vi "Logging Message Loop.vi"(8 "error in (no error)":errorcluster, 10 "Data Queue":refnum<queue>, 11 "Message Queues":T1) -> (0 "error out":errorcluster)   [LabVIEW 2017, in "Logging.lvlib"]
doc: "The message loop subVI to handle messages pertaining to logging data."
uses:
  Logging.lvlib
  support/Message Queue/All Message Queues.ctl
  support/Message Queue/Message Cluster.ctl
  Logging Configuration.ctl
  Logging State.ctl
  <userlib>/Circular Buffer/Controls/Circular Buffer Operations.ctl
  <userlib>/Circular Buffer/Instance VIs/Circular Buffer(2D Wfm with Attributes).vi
  support/Message Queue/Enqueue Message (Single).vi
  <vilib>/Waveform/WDTOps.llb/WDT Number of Waveform Samples DBL.vi
  <vilib>/Utility/error.llb/Error Cluster From Error Code.vi
  <vilib>/ErrorRing/Error Ring.xnode
  support/Message Queue/Message Queue.lvlib
  <userlib>/Circular Buffer/Circular Buffer.lvlib
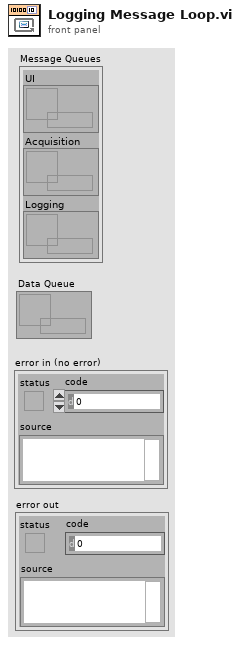
[diagram p1: front panel]
types:
  T1 = typedef "Message Queue.lvlib/All Message Queues.ctl" = cluster{"UI":refnum<queue>, "Acquisition":refnum<queue>, "Logging":refnum<queue>}
  T2 = typedef "Logging.lvlib/Logging State.ctl" = cluster{"State":enum16{"Logging", "Not Logging"}, "Samples to Save":u32, "Force Trigger":bool}
  T3 = typedef "Logging.lvlib/Logging Configuration.ctl" = cluster{"Log File Base Path":path, "Samples to Save":u32, "Trigger - Threshold":dbl, "Trigger - Channel":u32, "Always Log":bool, "External Trigger":bool, "External Trigger Armed":bool, "TDMS File Reference":refnum<k34>, "DAQVersion":string, "SWVersion":string, "CircSamples":u32, "BeepWhenComplete":bool, "ChannelConfig":string[][], "ActiveChannels":i32[], "Title":string, "Description":string, "ChannelNames":string[], "ResponseExtension":bool}
  T4 = typedef "Circular Buffer.lvlib/Circular Buffer Operations.ctl" = enum16{"Initialize", "Get Backlog", "Write", "Read (continuous)", "Read (most recent)", "Peak"}
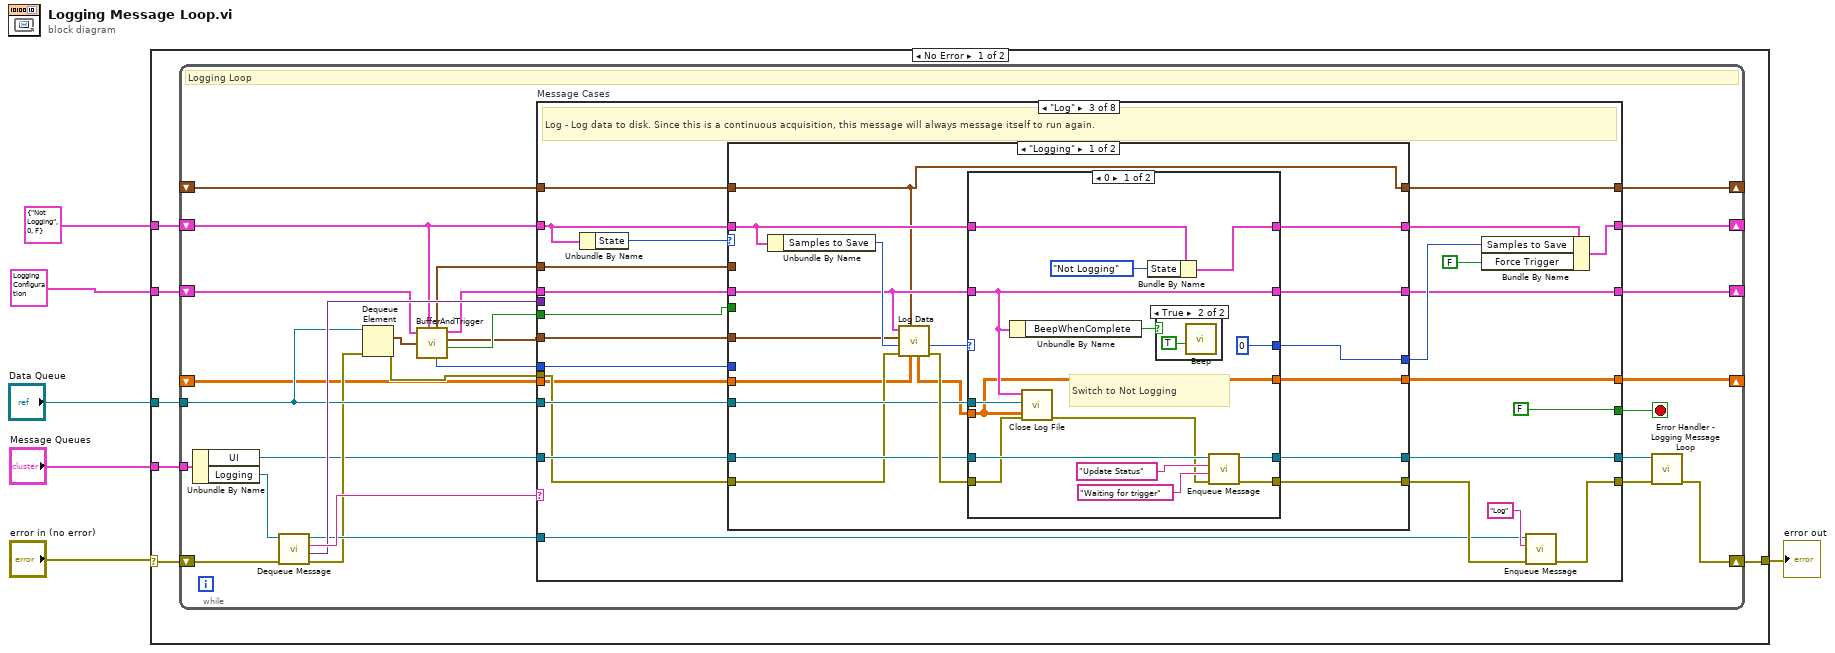
[diagram p0: block diagram]
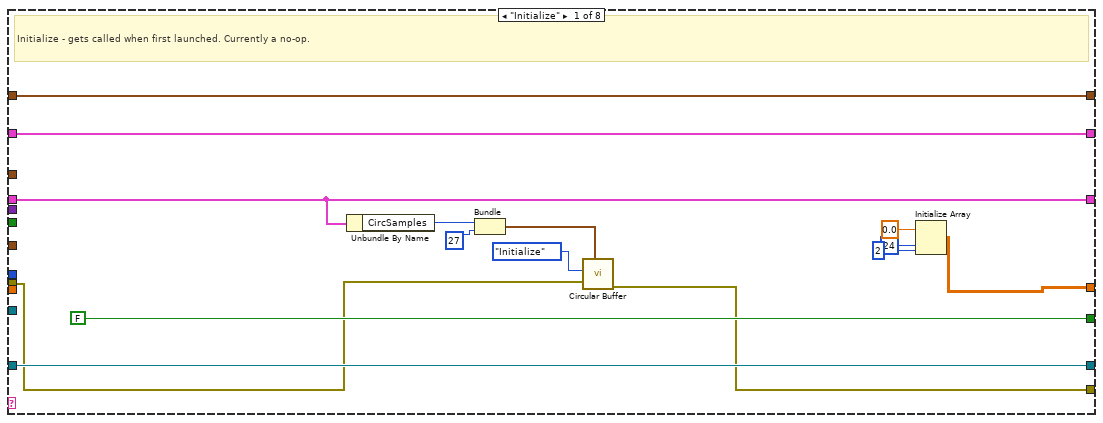
[diagram p2: hidden frame]
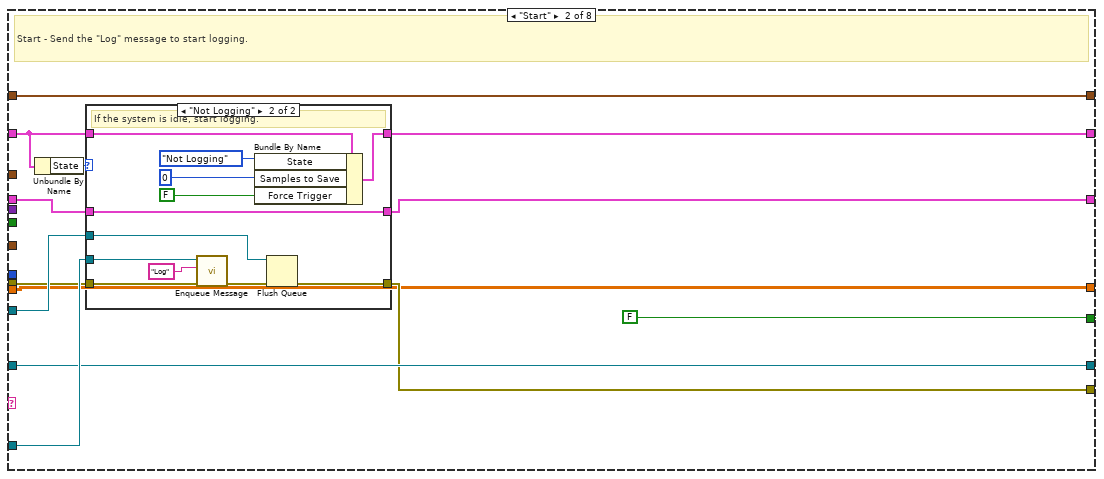
[diagram p3: hidden frame]
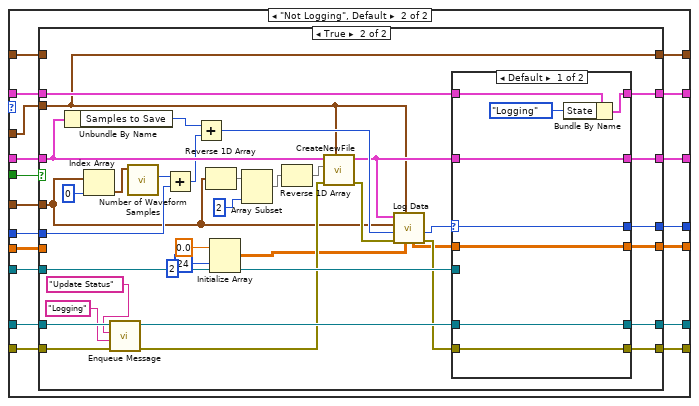
[diagram p7: hidden frame]
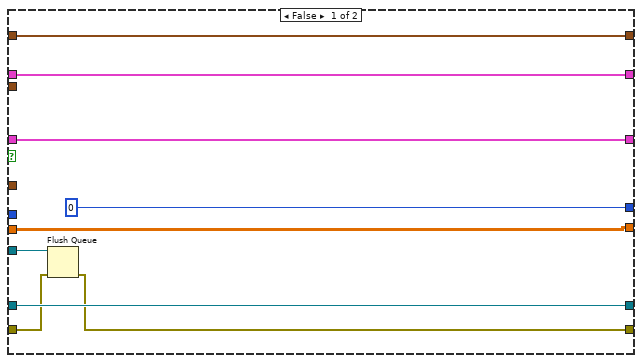
[diagram p8: hidden frame]
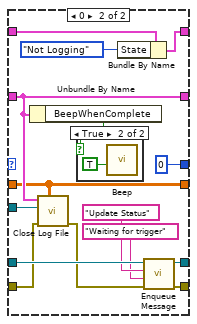
[diagram p9: hidden frame]
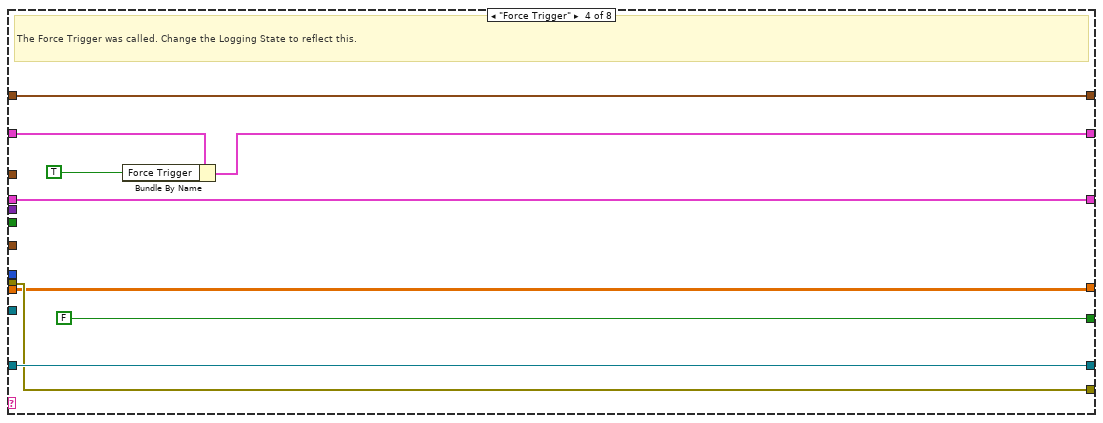
[diagram p11: hidden frame]
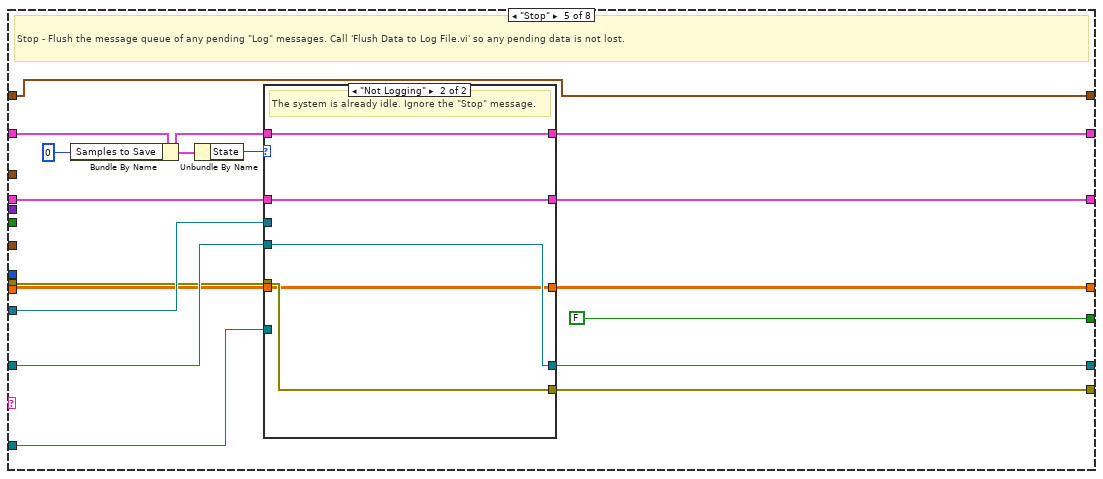
[diagram p12: hidden frame]
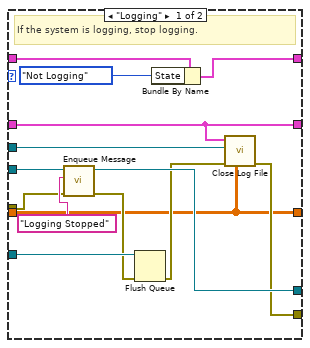
[diagram p13: hidden frame]
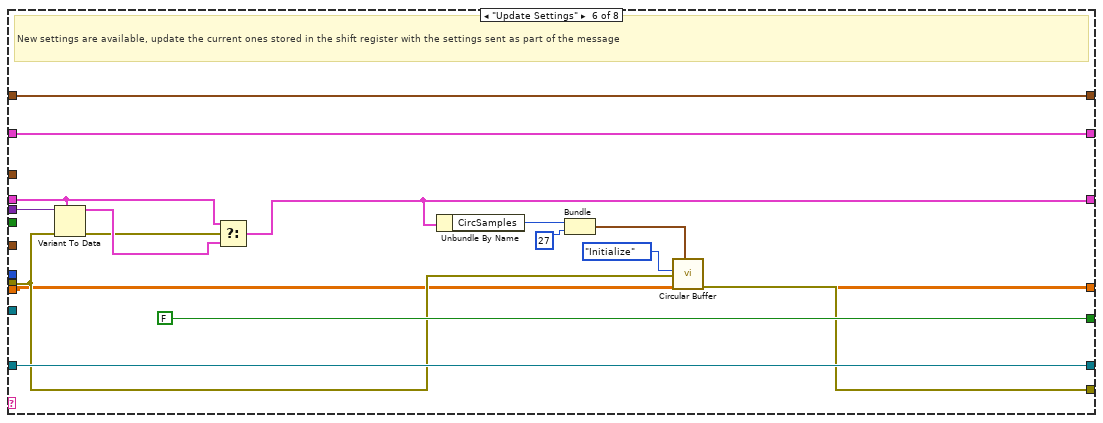
[diagram p14: hidden frame]
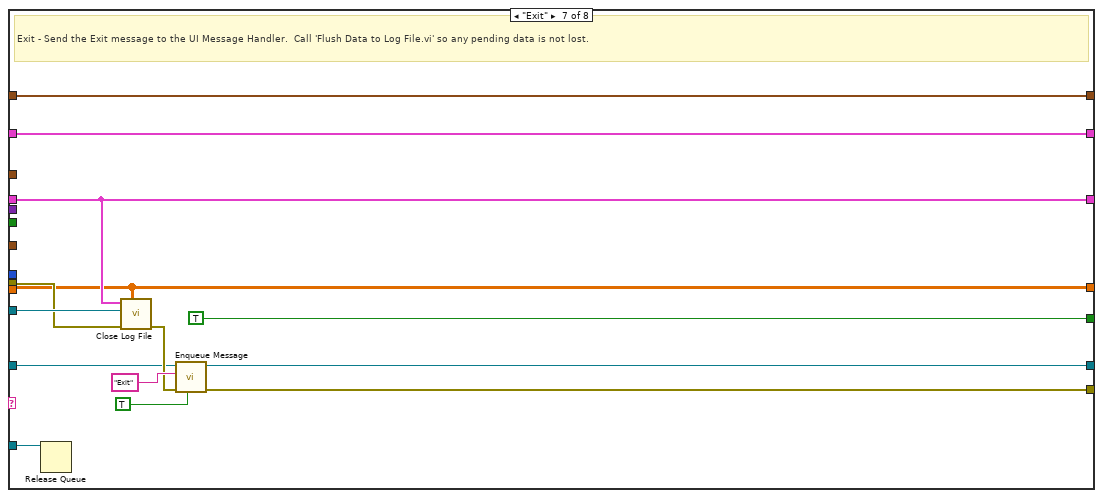
[diagram p15: hidden frame]
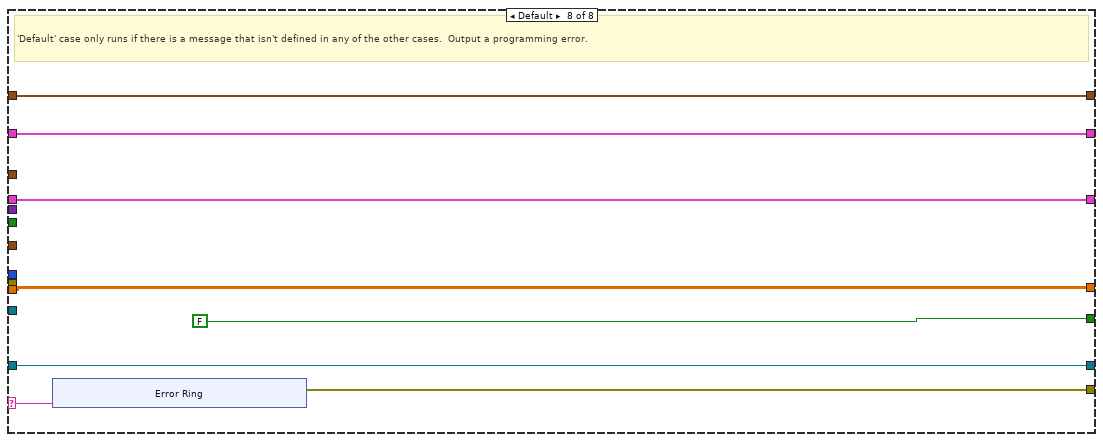
[diagram p16: hidden frame]
diagram:
  n1 = case shown="No Error" "error in (no error)" {
    selector: "error in (no error)" -> [w11 w327]
    tunnel: [w12 w327] -> w6
    tunnel: "Data Queue" -> [w10 _]
    tunnel: T2 {"State"=enum."Not Logging", "Samples to Save"=0, "Force Trigger"=FALSE} -> [w9 _]
    tunnel: T3 {"Log File Base Path"=path "", "Samples to Save"=0, "Trigger - Threshold"=0.0, "Trigger - Channel"=0, "Always Log"=FALSE, "External Trigger"=FALSE, "External Trigger Armed"=FALSE, "TDMS File Reference"=refnum, "DAQVersion"="", "SWVersion"="", "CircSamples"=0, "BeepWhenComplete"=FALSE, "ChannelConfig"=[], "ActiveChannels"=[], "Title"="", "Description"="", "ChannelNames"=[], "ResponseExtension"=TRUE} ("Logging Configuration") -> [w8 _]
    tunnel: "Message Queues" -> [w7 _]
    frame No Error {
      n2 = while {
        shift-right: [w32] -> w12
        shift-left: w11 -> [w31]
        tunnel: w10 -> [w35]
        shift-right: [w34] -> _
        shift-left: w9 -> [w21]
        tunnel: w7 -> [w27]
        shift-right: [w24] -> _
        shift-left: _ -> [w28]
        shift-right: [w40] -> _
        shift-left: w8 -> [w22]
        shift-right: [w13] -> _
        shift-left: _ -> [w14]
        stop <- w39 stop-if-true
        # "Logging Loop"
        n3 = Unbundle By Name(w27) -> ("UI"=w25:refnum<queue>, "Logging"=w26:refnum<queue>)
        n4 = call "Dequeue Message.vi"("error in (no error)"=w31, "Message Queue"=w26) -> ("error out"=w30:errorcluster, "Message Data"=w37:variant, "Message"=w38:string, "dup Message Queue"=w36:refnum<queue>)  [unwired: 6 in]
        n5 = Dequeue Element(queue=w35, error in (no error)=w30) -> (element=w23:waveform(dbl)[], error out=w15:errorcluster)  [unwired: 1 in, 2 out]
        n6 = call "BufferAndTrigger.vi"("Logging Configuration"=w22, "State"=w21, "WaveformIN"=w23) -> ("TriggerTimeStamp"=w18:timestamp, "Logging Configuration Out"=w20:T3, "WaveformOUT"=w17:waveform(dbl)[], "TriggerIndex"=w16:i32, "Trigger"=w19:bool)  [unwired: 2 in, 1 out]
        n7 = case "Message Cases" shown="\"Log\"" w38 {
          selector: w38 -> [_ _ _ _ _ _ _ w316]
          tunnel: w36 -> [_ w68 w95 _ w261 _ w308 _]
          tunnel: [w45 w58 w97 w239 w262 w284 w304 w317] -> w33
          tunnel: w20 -> [w47 w67 w93 w245 w256 w296 w307 w319]
          tunnel: [w47 w57 w100 w245 w255 w286 w307 w319] -> w40
          tunnel: [FALSE FALSE FALSE FALSE FALSE FALSE TRUE FALSE] -> w39
          tunnel: w37 -> [_ _ _ _ _ w297 _ _]
          tunnel: w25 -> [w54 w63 w98 w241 w259 w293 w303 w315]
          tunnel: w35 -> [_ w61 w99 _ w260 _ w301 _]
          tunnel: w21 -> [w55 w65 w106 w244 w252 w283 w306 w318]
          tunnel: [w55 w66 w105 w243 w257 w283 w306 w318] -> w34
          tunnel: w28 -> [w52 w59 w90 w238 w248 w291 w299 w313]
          tunnel: [w54 w63 w96 w241 w254 w293 w302 w315] -> w29
          tunnel: w17 -> [_ _ w92 _ _ _ _ _]
          tunnel: w15 -> [w46 w60 w91 w239 w249 w285 w300 _]
          tunnel: [w52 w59 w89 w238 w248 w291 w299 w313] -> w24
          tunnel: w19 -> [_ _ w88 _ _ _ _ _]
          tunnel: w18 -> [_ _ w87 _ _ _ _ _]
          tunnel: w16 -> [_ _ w86 _ _ _ _ _]
          tunnel: w14 -> [_ w56 w85 w237 w247 w282 w298 w312]
          tunnel: [w41 w56 w84 w237 w246 w282 w298 w312] -> w13
          frame "Initialize" {
            # "Initialize - gets called when first launched. Currently a no-op."
            n8 = Unbundle By Name(w47) -> ("CircSamples"=w50:u32)
            n9 = Bundle("CircSamples"=w50, 27) -> (w48:cluster{"CircSamples":u32, i32})  [unwired: 1 in]
            n10 = call-poly <userlib>:"Circular Buffer.vi"("Buffer Size"=w48, "error in (no error)"=w46, "Operation"=Circular_Buffer_Operations."Initialize") -> ("error out"=w45:errorcluster)  [unwired: 5 in, 3 out]
            n11 = Initialize Array(0.0 ("element"), 24 ("dimension size"), 2 ("dimension size")) -> (w41:dbl[][])
          }
          frame "Start" {
            # "Start - Send the \"Log\" message to start logging."
            n12 = Unbundle By Name(w65) -> ("State"=w64:enum16{"Logging", "Not Logging"})
            n13 = case shown="\"Not Logging\"" w64 {
              tunnel: [w69 w72] -> w58
              tunnel: w68 -> [_ w83]
              tunnel: w67 -> [w71 w73]
              tunnel: [w71 w73] -> w57
              tunnel: w65 -> [w70 w81]
              tunnel: [w70 w80] -> w66
              tunnel: w61 -> [_ w76]
              tunnel: w60 -> [w69 w74]
              frame "Logging", Default {
                # "The system is already running. Ignore the \"Start\" message."
              }
              frame "Not Logging" {
                # "If the system is idle, start logging."
                n14 = call-poly "Enqueue Message.vi"("error in (no error)"=w74, "Message"="Log", "Message Queue"=w83) -> ("error out"=w75:errorcluster)  [unwired: 7 in, 1 out]
                n15 = Bundle By Name(cluster=w81, "State"=enum16{"Logging", "Not Logging"}."Not Logging", "Samples to Save"=u32 0 ("Reads to Save"), "Force Trigger"=FALSE) -> (w80:T2)
                n16 = Flush Queue(queue=w76, error in (no error)=w75) -> (error out=w72:errorcluster)  [unwired: 2 out]
              }
            }
          }
          frame "Log" {
            # "Log - Log data to disk. Since this is a continuous acquisition, this message will always message itself to run again."
            n17 = Unbundle By Name(w106) -> ("State"=w107:enum16{"Logging", "Not Logging"})
            n18 = case shown="\"Logging\"" w107 {
              tunnel: [w124 w166] -> w103
              tunnel: w106 -> [w125 w161]
              tunnel: w98 -> [w120 w165]
              tunnel: [w121 w155] -> w101
              tunnel: [w123 w164] -> w102
              tunnel: [w118 w163] -> w100
              tunnel: w99 -> [w119 w162]
              tunnel: w90 -> [w112 w152]
              tunnel: [w116 w160] -> w96
              tunnel: w92 -> [w113 w159]
              tunnel: w91 -> [w114 w157]
              tunnel: w88 -> [_ w156]
              tunnel: w93 -> [w115 w158]
              tunnel: [w112 w154] -> w89
              tunnel: w87 -> [_ w153]
              tunnel: w86 -> [_ w151]
              tunnel: w85 -> [w111 w150]
              tunnel: [w109 w149] -> w84
              frame "Logging" {
                n19 = Unbundle By Name(w125) -> ("Samples to Save"=w126:u32)
                n20 = call "Log Data.vi"("MinMax_in"=w111, "TriggerTimeStamp"=w112, "error in (no error)"=w114, "Samples to Save In"=w126, "Data"=w113, "Logging Configuration"=w115) -> ("error out"=w122:errorcluster, "Samples to Save Out"=w117:u32, "MinMax_out"=w110:dbl[][])  [unwired: 3 in]
                n21 = case shown="0" w117 {
                  selector: w117 -> [_ w148]
                  tunnel: w122 -> [w134 w147]
                  tunnel: [w138 w147] -> w121
                  tunnel: w125 -> [w140 w146]
                  tunnel: [w139 w146] -> w124
                  tunnel: [u32 0 ("Samples to Save Out") w148] -> w123
                  tunnel: w120 -> [w135 w144]
                  tunnel: w119 -> [w130 _]
                  tunnel: w115 -> [w129 w145]
                  tunnel: [w129 w145] -> w118
                  tunnel: [w132 w144] -> w116
                  tunnel: w110 -> [w127 w143]
                  tunnel: [w127 w143] -> w109
                  frame 0 {
                    # "Switch to Not Logging"
                    n22 = Unbundle By Name(w129) -> ("BeepWhenComplete"=w128:bool)
                    n23 = call "Close Log File.vi"("MinMax_in"=w127, "error in (no error)"=w134, "Data Queue"=w130, "Logging Configuration"=w129) -> ("error out"=w133:errorcluster)  [unwired: 7 in]
                    n24 = Bundle By Name(cluster=w140, "State"=enum16{"Logging", "Not Logging"}."Not Logging") -> (w139:T2)
                    n25 = case shown="True" w128 {
                      frame False {
                      }
                      frame True {
                        n26 = call <vilib>:"Beep.vi"("use system alert? (T)"=TRUE) -> ()  [unwired: 11 in]
                      }
                    }
                    n27 = call-poly "Enqueue Message.vi"("error in (no error)"=w133, "Message Data"="Waiting for trigger" ("Waiting for trigger"), "Message"="Update Status", "Message Queue"=w135) -> ("error out"=w138:errorcluster, "dup Message Queue"=w132:refnum<queue>)  [unwired: 6 in]
                  }
                  frame Default {
                    # "Continue in our same State."
                  }
                }
              }
              frame "Not Logging", Default {
                n28 = case shown="True" w156 {
                  tunnel: w157 -> [w171 w201]
                  tunnel: w158 -> [w174 w196]
                  tunnel: w161 -> [w175 w208]
                  tunnel: [w175 w207] -> w166
                  tunnel: w165 -> [w173 w212]
                  tunnel: [u32 0 ("Samples to Save Out") w209] -> w164
                  tunnel: [w174 w205] -> w163
                  tunnel: w152 -> [w168 _]
                  tunnel: w162 -> [w172 w203]
                  tunnel: [w173 w204] -> w160
                  tunnel: w159 -> [_ w186]
                  tunnel: [w169 w200] -> w155
                  tunnel: [w168 w192] -> w154
                  tunnel: w153 -> [_ w192]
                  tunnel: w151 -> [_ w188]
                  tunnel: w150 -> [w167 _]
                  tunnel: [w167 w176] -> w149
                  frame False {
                    n29 = Flush Queue(queue=w172, error in (no error)=w171) -> (error out=w169:errorcluster)  [unwired: 2 out]
                  }
                  frame True {
                    n30 = Unbundle By Name(w196) -> ("Samples to Save"=w198:u32)
                    n31 = Index Array(array=w186, index=0) -> (element=w191:waveform(dbl))
                    n32 = call-poly "Enqueue Message.vi"("error in (no error)"=w201, "Message Data"="Logging" ("Logging"), "Message"="Update Status", "Message Queue"=w212) -> ("error out"=w194:errorcluster, "dup Message Queue"=w206:refnum<queue>)  [unwired: 6 in]
                    n33 = call-poly <vilib>:"Number of Waveform Samples.vi"("waveform in"=w191) -> ("number of samples"=w189:i32)  [unwired: 8 in, 2 out]
                    n34 = Add(x=w189, y=w188) -> (x+y=w187:i32)
                    n35 = Add(x=w198, y=w187) -> (x+y=w199:u32)
                    n36 = Reverse 1D Array(array=w186) -> (reversed array=w185:waveform(dbl)[])
                    n37 = Initialize Array(0.0 ("element"), 24 ("dimension size"), 2 ("dimension size")) -> (w181:dbl[][])
                    n38 = Array Subset(array=w185, length=2) -> (w183:waveform(dbl)[])  [unwired: 1 in]
                    n39 = Reverse 1D Array(array=w183) -> (reversed array=w182:waveform(dbl)[])
                    n40 = call "CreateNewFile.vi"("TriggerTimeStamp"=w192, "error in (no error)"=w194, "Data"=w182, "Logging Configuration"=w196) -> ("error out"=w193:errorcluster, "Logging Config Out"=w195:T3)  [unwired: 6 in]
                    n41 = call "Log Data.vi"("MinMax_in"=w181, "TriggerTimeStamp"=w192, "error in (no error)"=w193, "Samples to Save In"=w199, "Data"=w186, "Logging Configuration"=w195) -> ("error out"=w202:errorcluster, "Samples to Save Out"=w197:u32, "MinMax_out"=w177:dbl[][])  [unwired: 3 in]
                    n42 = case shown="Default" w197 {
                      selector: w197 -> [w220 _]
                      tunnel: [w220 u32 0 ("Samples to Save Out")] -> w209
                      tunnel: [w217 w226] -> w207
                      tunnel: w208 -> [w218 w227]
                      tunnel: w202 -> [w216 w225]
                      tunnel: [w216 w232] -> w200
                      tunnel: w206 -> [w214 w235]
                      tunnel: w195 -> [w215 w223]
                      tunnel: [w215 w223] -> w205
                      tunnel: [w214 w231] -> w204
                      tunnel: w203 -> [_ w229]
                      tunnel: w177 -> [w213 w221]
                      tunnel: [w213 w221] -> w176
                      frame Default {
                        n43 = Bundle By Name(cluster=w218, "State"=enum16{"Logging", "Not Logging"}."Logging") -> (w217:T2)
                      }
                      frame 0 {
                        n44 = Unbundle By Name(w223) -> ("BeepWhenComplete"=w222:bool)
                        n45 = call "Close Log File.vi"("MinMax_in"=w221, "error in (no error)"=w225, "Data Queue"=w229, "Logging Configuration"=w223) -> ("error out"=w224:errorcluster)  [unwired: 7 in]
                        n46 = case shown="True" w222 {
                          frame False {
                          }
                          frame True {
                            n47 = call <vilib>:"Beep.vi"("use system alert? (T)"=TRUE) -> ()  [unwired: 11 in]
                          }
                        }
                        n48 = Bundle By Name(cluster=w227, "State"=enum16{"Logging", "Not Logging"}."Not Logging") -> (w226:T2)
                        n49 = call-poly "Enqueue Message.vi"("error in (no error)"=w224, "Message Data"="Waiting for trigger" ("Waiting for trigger"), "Message"="Update Status", "Message Queue"=w235) -> ("error out"=w232:errorcluster, "dup Message Queue"=w231:refnum<queue>)  [unwired: 6 in]
                      }
                    }
                  }
                }
              }
            }
            n50 = Bundle By Name(cluster=w103, "Samples to Save"=w102, "Force Trigger"=FALSE) -> (w105:T2)
            n51 = call-poly "Enqueue Message.vi"("error in (no error)"=w101, "Message"="Log", "Message Queue"=w95) -> ("error out"=w97:errorcluster)  [unwired: 7 in, 1 out]
          }
          frame "Force Trigger" {
            # "The Force Trigger was called. Change the Logging State to reflect this."
            n52 = Bundle By Name(cluster=w244, "Force Trigger"=TRUE) -> (w243:T2)
          }
          frame "Stop" {
            # "Stop - Flush the message queue of any pending \"Log\" messages. Call 'Flush Data to Log File.vi' so any pending data is not lost."
            n53 = Bundle By Name(cluster=w252, "Samples to Save"=u32 0) -> (w250:T2)
            n54 = Unbundle By Name(w250) -> ("State"=w258:enum16{"Logging", "Not Logging"})
            n55 = case shown="\"Not Logging\"" w258 {
              tunnel: [w268 w281] -> w262
              tunnel: w249 -> [w265 w281]
              tunnel: w261 -> [w276 _]
              tunnel: w256 -> [w270 w279]
              tunnel: w260 -> [w267 _]
              tunnel: w259 -> [w271 w278]
              tunnel: w250 -> [w274 w280]
              tunnel: [w273 w280] -> w257
              tunnel: [w270 w279] -> w255
              tunnel: [w269 w278] -> w254
              tunnel: w247 -> [w263 w277]
              tunnel: [w263 w277] -> w246
              frame "Logging" {
                # "If the system is logging, stop logging."
                n56 = call-poly "Enqueue Message.vi"("error in (no error)"=w265, "Message"="Logging Stopped", "Message Queue"=w271) -> ("error out"=w264:errorcluster, "dup Message Queue"=w269:refnum<queue>)  [unwired: 7 in]
                n57 = Flush Queue(queue=w276, error in (no error)=w264) -> (error out=w266:errorcluster)  [unwired: 2 out]
                n58 = Bundle By Name(cluster=w274, "State"=enum16{"Logging", "Not Logging", "Idle"}."Not Logging") -> (w273:T2)
                n59 = call "Close Log File.vi"("MinMax_in"=w263, "error in (no error)"=w266, "Data Queue"=w267, "Logging Configuration"=w270) -> ("error out"=w268:errorcluster)  [unwired: 7 in]
              }
              frame "Not Logging" {
                # "The system is already idle. Ignore the \"Stop\" message."
              }
            }
          }
          frame "Update Settings" {
            # "New settings are available, update the current ones stored in the shift register with the settings sent as part of the message"
            n60 = Variant To Data(error in=w285, type=w296, Variant=w297) -> (data=w295:T3, error out=w294:errorcluster)
            n61 = Select(t=w296, s=w294, f=w295) -> (s? t:f=w286:T3)
            n62 = Unbundle By Name(w286) -> ("CircSamples"=w289:u32)
            n63 = Bundle("CircSamples"=w289, 27) -> (w287:cluster{"CircSamples":u32, i32})  [unwired: 1 in]
            n64 = call-poly <userlib>:"Circular Buffer.vi"("Buffer Size"=w287, "error in (no error)"=w285, "Operation"=Circular_Buffer_Operations."Initialize") -> ("error out"=w284:errorcluster)  [unwired: 5 in, 3 out]
          }
          frame "Exit" {
            # "Exit - Send the Exit message to the UI Message Handler.  Call 'Flush Data to Log File.vi' so any pending data is not lost."
            n65 = Release Queue(queue=w308) -> ()  [unwired: 2 in, 3 out]
            n66 = call "Close Log File.vi"("MinMax_in"=w298, "error in (no error)"=w300, "Data Queue"=w301, "Logging Configuration"=w307) -> ("error out"=w305:errorcluster)  [unwired: 7 in]
            n67 = call-poly "Enqueue Message.vi"("Priority Message? (F)"=TRUE, "error in (no error)"=w305, "Message"="Exit", "Message Queue"=w303) -> ("error out"=w304:errorcluster, "dup Message Queue"=w302:refnum<queue>)  [unwired: 6 in]
          }
          frame Default {
            # "'Default' case only runs if there is a message that isn't defined in any of the other cases.  Output a programming error."
            n68 = xnode "Error Ring"("parameter 0"=w316) -> ("error out"=w317:errorcluster)
          }
        }
        n69 = call "Error Handler - Logging Message Loop.vi"("error in (no error)"=w33, "Message Queue"=w29) -> ("dup error in"=w32:errorcluster)  [unwired: 8 in, 1 out]
      }
    }
    frame Error {
    }
  }
  "error out" <- w6
